vi "OpenScanFile.vi"(8 "error in":errorcluster) -> (0 "error out":errorcluster, 3 "refnum out":refnum<file>)   [LabVIEW 2012]
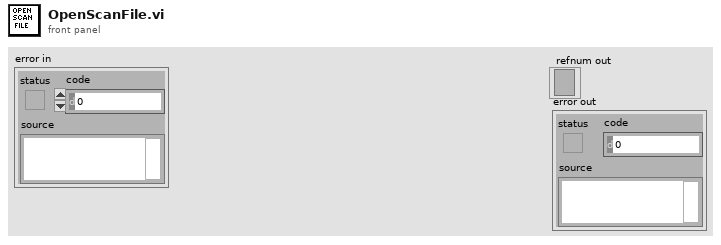
[diagram p1: front panel]
types:
  T1 = enum16{"open", "replace", "create", "open or create", "replace or create", "replace or create with confirmation"}
  T2 = enum16{"deny read/write", "deny write-only", "deny none"}
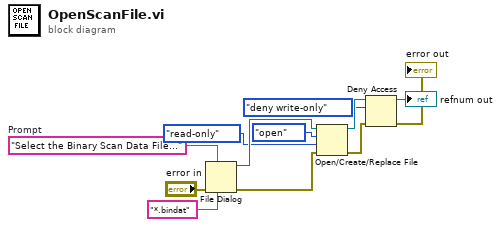
[diagram p0: block diagram]
diagram:
  w11 = "Select the Binary Scan Data File..."  # Prompt
  n1 = File Dialog(6:"*.bindat" ("pattern (all files)"), 7:w11, 8:"error in") -> (0:w9:errorcluster, 3:w12:path)  [unwired: 4 in, 2 out]
  n2 = Open/Create/Replace File(file path (use dialog)=w12, error in=w9, operation (0:open)=T1."open", access (0:read/write)=enum16{"read/write", "read-only", "write-only"}."read-only") -> (refnum out=w6:refnum<file>, error out=w7:errorcluster)  [unwired: 2 in, 1 out]
  n3 = Deny Access(4:w7, 6:T2."deny write-only" ("deny mode (0:deny read/write)"), 7:w6) -> (0:→"error out":errorcluster, 3:→"refnum out":refnum<file>)
